vi "tm3samp_06_framerate.vi"() -> ()   [LabVIEW 2023]
panel:
  out "Software FPS":dbl
  out "Camera FPS":dbl
  out "Image":u16[][](graph)
  out "Camera Serial":string
  out "Camera Version":string
  out "Camera Model":string
  out "SMD":dbl
  in  "Scan Mode":dbl min=1.0 max=2.0 step=1.0
  in  "Exposure":dbl min=0.0030207518796992482 max=10.0 step=9.999999747378752e-06
  out "EXP":dbl
  out "SVW":i32
  out "SHW":i32
  out "SVO":i32
  out "SHO":i32
  in  "V Width":i32 min=4 max=2048 step=4
  in  "V Offset":i32 min=0 max=1024 step=4
  in  "H Width":i32 min=4 max=2048 step=4
  in  "H Offset":i32 min=0 max=0 step=4
  in  "Binning":u16(ring) items=["1x1"=1, "2x2"=2, "4x4"=4]
  out "Elapsed Time":u32
  out "Total Frames":i32
  in  "Display":bool=TRUE
  out "error out":errorcluster
  in  "stop":bool
  # "This example displays the frame rate\nof the camera.  Changing the resolution\nof the camera or displaying the images\nwill affect the frame rate."
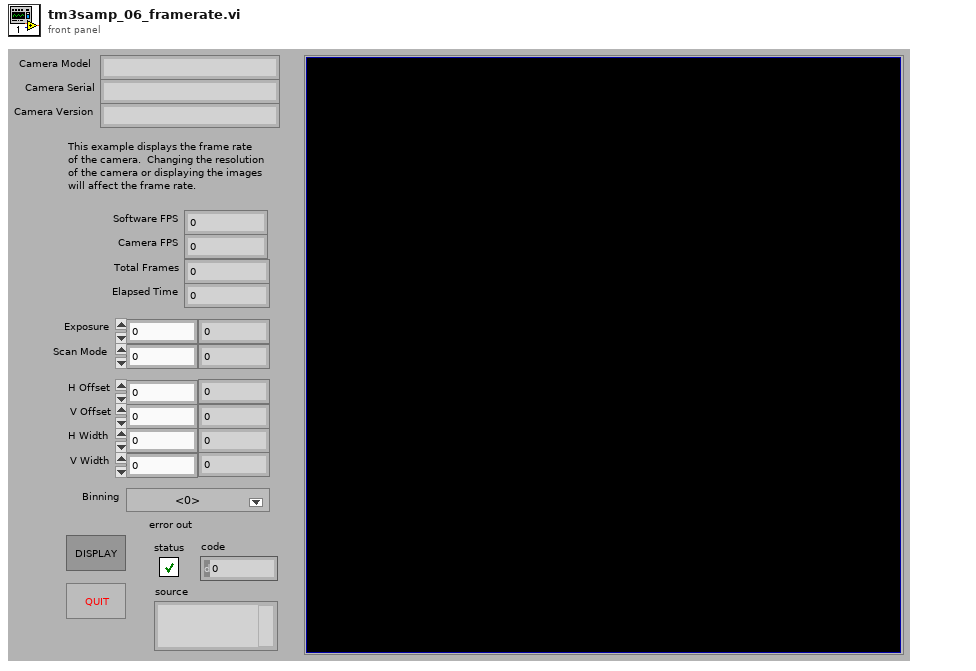
[diagram p1: front panel]
types:
  T1 = cluster{"Model":string, "Camera ID":string, "Firmware":string}
  T2 = cluster{"Value":i32, "Minimum":i32, "Maximum":i32, "Increment":i32}
  T3 = cluster{"height":u32, "width":u32, "datatype":u32}
  T4 = cluster{"H Offset":i32, "V Offset":i32, "H Width":i32, "V Width":i32}
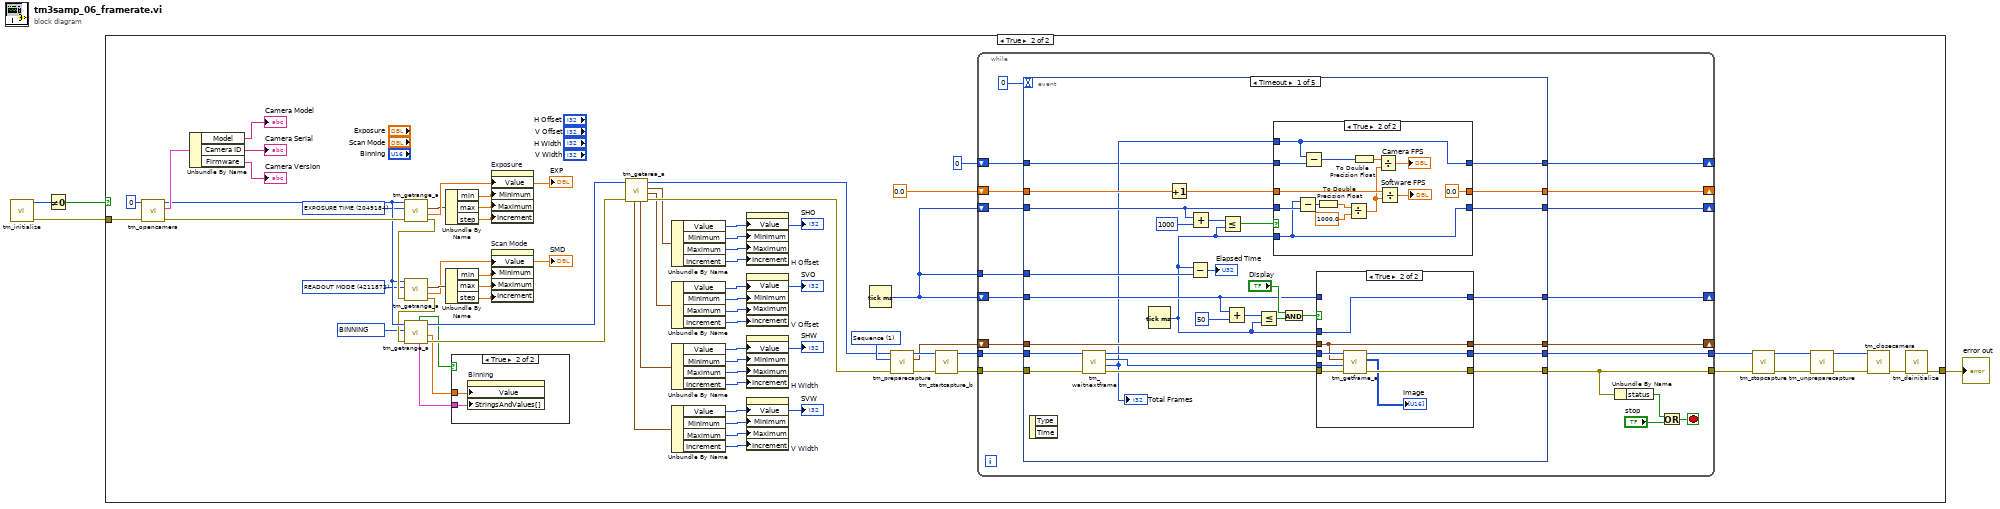
[diagram p0: block diagram]
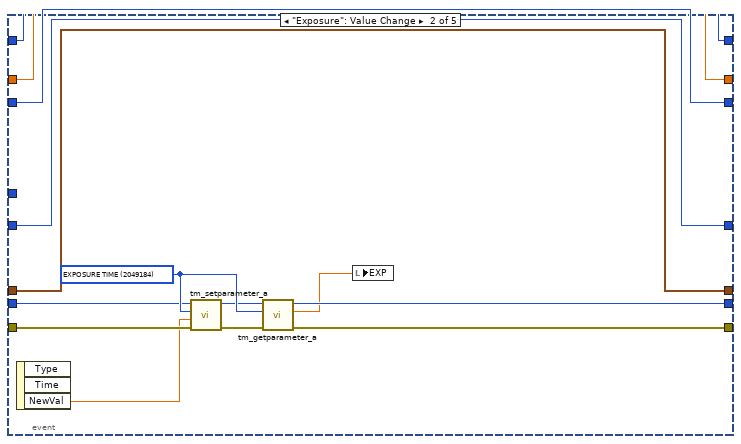
[diagram p6: hidden frame]
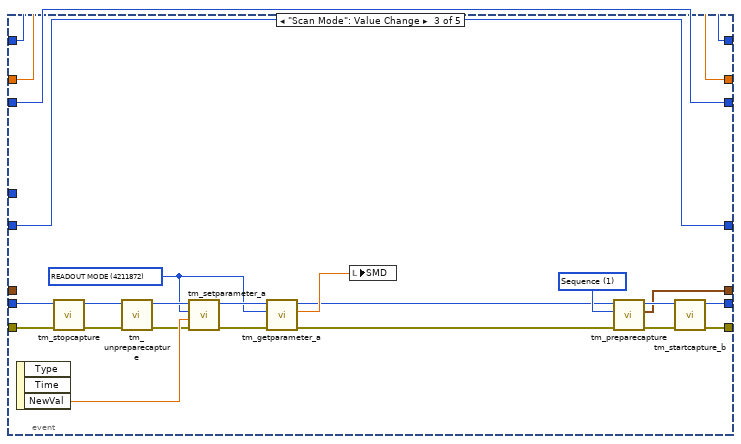
[diagram p7: hidden frame]
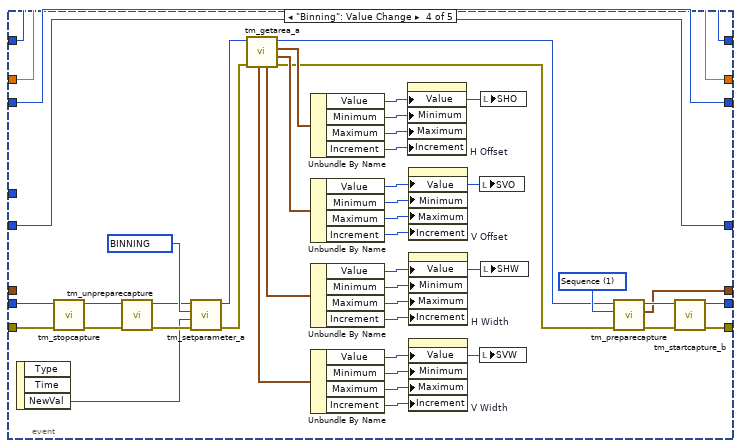
[diagram p8: hidden frame]
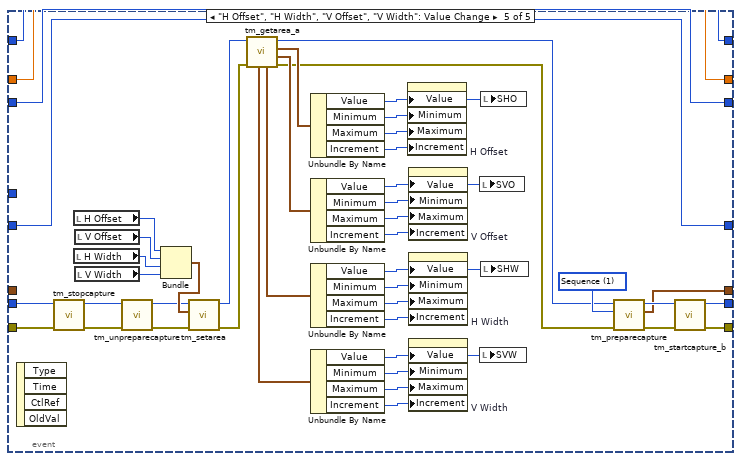
[diagram p9: hidden frame]
diagram:
  n1 = call "tm_initialize.vi"() -> ("error out"=w2:errorcluster, "Number Of Cameras"=w1:u32)  [unwired: 8 in, 2 out]
  n2 = Not Equal To 0?(x=w1) -> (x != 0?=w4:bool)
  n3 = case shown="True" w4 {
    tunnel: [w5 w69] -> w3
    tunnel: w2 -> [w5 w72]
    frame False {
    }
    frame True {
      w6 = u32 2049184 items=["BINNING"=4215968, "BITS PER CHANNEL"=4342976, "ACTIVE VIEW INDEX"=4343136, "CCD MODE"=4212384, "SENSOR MODE"=4212128, "READOUT MODE"=4211872, "EXPOSURE TIME"=2049184, "CONTRAST GAIN"=3163312, "CONTRAST OFFSET"=3163328, "LIGHT MODE"=2114720, "SENSITIVITY"=2114992, "WHITE BALANCE"=3163568, "PHOTON IMAGING MODE"=2115200, "HIGH DYNAMIC RANGE MODE"=3163360, "TRIGGER SOURCE"=1066144, "TRIGGER ACTIVE"=1066160, "TRIGGER MODE"=1066400, "TRIGGER POLARITY"=1066416, "TRIGGER GLOBAL EXPOSURE"=2049680, "FIRST TRIGGER BEHAVIOR"=2049696, "TRIGGER TIMES"=1066448, "OUTPUT TRIGGER POLARITY"=1852592, "OUTPUT TRIGGER DELAY"=1852624, "OUTPUT TRIGGER PERIOD"=1852640, "TEMPERATURE"=2115232, "TEMPERATURE TARGET"=2115264, "SENSOR COOLER FAN"=2115296, "MECHANICAL SHUTTER"=2115488, "BACK FOCUS POSITION"=8422304, "FRAMEBUNDLE MODE"=4346784, "FRAMEBUNDLE NUMBER"=4346800, "LINEBUNDLE HEIGHT"=4212192, "TRIGGER CONNECTOR"=1066432, "IMAGE PIXEL TYPE"=4343296, "OUTPUT TRIGGER KIND"=1852656, "READOUT DIRECTION"=4211904, "CHANNEL SYNC"=1852352] ("Parameter")
      w7 = u32 4211872 items=["BINNING"=4215968, "BITS PER CHANNEL"=4342976, "ACTIVE VIEW INDEX"=4343136, "CCD MODE"=4212384, "SENSOR MODE"=4212128, "READOUT MODE"=4211872, "EXPOSURE TIME"=2049184, "CONTRAST GAIN"=3163312, "CONTRAST OFFSET"=3163328, "LIGHT MODE"=2114720, "SENSITIVITY"=2114992, "WHITE BALANCE"=3163568, "PHOTON IMAGING MODE"=2115200, "HIGH DYNAMIC RANGE MODE"=3163360, "TRIGGER SOURCE"=1066144, "TRIGGER ACTIVE"=1066160, "TRIGGER MODE"=1066400, "TRIGGER POLARITY"=1066416, "TRIGGER GLOBAL EXPOSURE"=2049680, "FIRST TRIGGER BEHAVIOR"=2049696, "TRIGGER TIMES"=1066448, "OUTPUT TRIGGER POLARITY"=1852592, "OUTPUT TRIGGER DELAY"=1852624, "OUTPUT TRIGGER PERIOD"=1852640, "TEMPERATURE"=2115232, "TEMPERATURE TARGET"=2115264, "SENSOR COOLER FAN"=2115296, "MECHANICAL SHUTTER"=2115488, "BACK FOCUS POSITION"=8422304, "FRAMEBUNDLE MODE"=4346784, "FRAMEBUNDLE NUMBER"=4346800, "LINEBUNDLE HEIGHT"=4212192, "TRIGGER CONNECTOR"=1066432, "IMAGE PIXEL TYPE"=4343296, "OUTPUT TRIGGER KIND"=1852656, "READOUT DIRECTION"=4211904, "CHANNEL SYNC"=1852352] ("Parameter")
      w8 = u32 4215968 items=["BINNING"=4215968, "BITS PER CHANNEL"=4342976, "ACTIVE VIEW INDEX"=4343136, "CCD MODE"=4212384, "SENSOR MODE"=4212128, "READOUT MODE"=4211872, "EXPOSURE TIME"=2049184, "CONTRAST GAIN"=3163312, "CONTRAST OFFSET"=3163328, "LIGHT MODE"=2114720, "SENSITIVITY"=2114992, "WHITE BALANCE"=3163568, "PHOTON IMAGING MODE"=2115200, "HIGH DYNAMIC RANGE MODE"=3163360, "TRIGGER SOURCE"=1066144, "TRIGGER ACTIVE"=1066160, "TRIGGER MODE"=1066400, "TRIGGER POLARITY"=1066416, "TRIGGER GLOBAL EXPOSURE"=2049680, "FIRST TRIGGER BEHAVIOR"=2049696, "TRIGGER TIMES"=1066448, "OUTPUT TRIGGER POLARITY"=1852592, "OUTPUT TRIGGER DELAY"=1852624, "OUTPUT TRIGGER PERIOD"=1852640, "TEMPERATURE"=2115232, "TEMPERATURE TARGET"=2115264, "SENSOR COOLER FAN"=2115296, "MECHANICAL SHUTTER"=2115488, "BACK FOCUS POSITION"=8422304, "FRAMEBUNDLE MODE"=4346784, "FRAMEBUNDLE NUMBER"=4346800, "LINEBUNDLE HEIGHT"=4212192, "TRIGGER CONNECTOR"=1066432, "IMAGE PIXEL TYPE"=4343296, "OUTPUT TRIGGER KIND"=1852656, "READOUT DIRECTION"=4211904, "CHANNEL SYNC"=1852352] ("Parameter")
      w67 = 1 items=["Snap", "Sequence"] ("Capture mode")
      n4 = call "tm_opencamera.vi"("error in (no error)"=w72, "Camera Index"=u32 0) -> ("error out"=w21:errorcluster, "Camera Details"=w25:T1, "Handle out"=w15:u32)  [unwired: 7 in]
      n5 = Unbundle By Name(w25) -> ("Model"=→"Camera Model":string, "Camera ID"=→"Camera Serial":string, "Firmware"=→"Camera Version":string)
      n6 = call "tm_getrange_a.vi"("error in (no error)"=w21, "Parameter"=w6, "Handle in"=w15) -> ("error out"=w18:errorcluster, "default"=w20:dbl, "Range"=w19:cluster{"min":dbl, "max":dbl, "step":dbl})  [unwired: 2 in, 4 out]
      "EXP" <- w20
      n7 = call "tm_getrange_a.vi"("error in (no error)"=w18, "Parameter"=w7, "Handle in"=w15) -> ("error out"=w14:errorcluster, "default"=w16:dbl, "Range"=w17:cluster{"min":dbl, "max":dbl, "step":dbl})  [unwired: 2 in, 4 out]
      "SMD" <- w16
      n8 = call "tm_getrange_a.vi"("error in (no error)"=w14, "Parameter"=w8, "Handle in"=w15) -> ("error out"=w13:errorcluster, "default"=w10:dbl, "Handle out"=w12:u32, "Value Names"=w9:cluster{"Name":string, "Value":dbl}[], "Writable"=w11:bool)  [unwired: 2 in, 2 out]
      n9 = Unbundle By Name(w19) -> ("min"=w60:dbl, "max"=w59:dbl, "step"=w58:dbl)
      n10 = Unbundle By Name(w17) -> ("min"=w57:dbl, "max"=w56:dbl, "step"=w55:dbl)
      n11 = case shown="True" w11 {
        tunnel: w9 -> [_ w74]
        tunnel: w10 -> [_ w73]
        frame False {
        }
        frame True {
          n12 = property on="Binning" class="Ring (strict)"("Value"=w73, "StringsAndValues[]"=w74) -> ()  [unwired: 2 in, 2 out]
        }
      }
      n13 = property on="Exposure" class="DigNum (strict)"("Value"=w20, "Minimum"=w60, "Maximum"=w59, "Increment"=w58) -> ()  [unwired: 2 in, 2 out]
      n14 = property on="Scan Mode" class="DigNum (strict)"("Value"=w16, "Minimum"=w57, "Maximum"=w56, "Increment"=w55) -> ()  [unwired: 2 in, 2 out]
      n15 = call "tm_getarea_a.vi"("error in (no error)"=w13, "Handle in"=w12) -> ("error out"=w53:errorcluster, "V Offset"=w52:T2, "H Offset"=w31:T2, "Handle out"=w54:u32, "H Width"=w51:T2, "V Width"=w50:T2)  [unwired: 4 in]
      n16 = Unbundle By Name(w31) -> ("Value"=w30:i32, "Minimum"=w29:i32, "Maximum"=w28:i32, "Increment"=w27:i32)
      "SHO" <- w30
      n17 = Unbundle By Name(w52) -> ("Value"=w40:i32, "Minimum"=w49:i32, "Maximum"=w48:i32, "Increment"=w47:i32)
      "SVO" <- w40
      n18 = Unbundle By Name(w51) -> ("Value"=w39:i32, "Minimum"=w46:i32, "Maximum"=w45:i32, "Increment"=w44:i32)
      "SHW" <- w39
      n19 = Unbundle By Name(w50) -> ("Value"=w38:i32, "Minimum"=w43:i32, "Maximum"=w42:i32, "Increment"=w41:i32)
      "SVW" <- w38
      n20 = property on="H Offset" class="DigNum (strict)"("Value"=w30, "Minimum"=w29, "Maximum"=w28, "Increment"=w27) -> ()  [unwired: 2 in, 2 out]
      n21 = property on="V Offset" class="DigNum (strict)"("Value"=w40, "Minimum"=w49, "Maximum"=w48, "Increment"=w47) -> ()  [unwired: 2 in, 2 out]
      n22 = property on="H Width" class="DigNum (strict)"("Value"=w39, "Minimum"=w46, "Maximum"=w45, "Increment"=w44) -> ()  [unwired: 2 in, 2 out]
      n23 = property on="V Width" class="DigNum (strict)"("Value"=w38, "Minimum"=w43, "Maximum"=w42, "Increment"=w41) -> ()  [unwired: 2 in, 2 out]
      n24 = Tick Count (ms)() -> (millisecond timer value=w61:u32)
      n25 = call "tm_preparecapture.vi"("error in (no error)"=w53, "Capture mode"=w67, "Handle in"=w54) -> ("error out"=w65:errorcluster, "Buffer Info"=w62:T3, "Handle out"=w66:u32)  [unwired: 5 in, 1 out]
      n26 = call "tm_startcapture_b.vi"("error in (no error)"=w65, "Handle in"=w66) -> ("error out"=w64:errorcluster, "Handle out"=w63:u32)  [unwired: 8 in]
      n27 = while {
        tunnel: w64 -> [w82]
        tunnel: [w80] -> w37
        tunnel: [w79] -> w36
        shift-right: [w89] -> _
        shift-left: w61 -> [w87]
        shift-right: [w90] -> _
        shift-left: 0.0 -> [w88]
        shift-right: [w81] -> _
        shift-left: w61 -> [w85]
        tunnel: w63 -> [w83]
        tunnel: w61 -> [w86]
        shift-right: [w78] -> _
        shift-left: w62 -> [w84]
        shift-right: [w75] -> _
        shift-left: 0 -> [w76]
        stop <- w91 stop-if-true
        n28 = event shown="[0] Timeout" {
          selector: _ -> [_ _ _ _ _]
          dyn-events: _ -> [_ _ _ _ _]
          timeout: 0 -> [_ _ _ _ _]
          tunnel: [w98 w164 w187 w223 w268] -> w90
          tunnel: [w97 w165 w188 w224 w269] -> w89
          tunnel: w88 -> [w109 w164 w187 w223 w268]
          tunnel: w87 -> [w100 w165 w188 w224 w269]
          tunnel: w86 -> [w105 _ _ _ _]
          tunnel: w85 -> [w110 w166 w189 w231 w276]
          tunnel: w84 -> [w104 w163 _ _ _]
          tunnel: w83 -> [w112 w158 w184 w200 w238]
          tunnel: w82 -> [w111 w160 w183 w199 w237]
          tunnel: [w108 w166 w189 w231 w276] -> w81
          tunnel: [w107 w155 w178 w226 w271] -> w80
          tunnel: [w106 w153 w179 w227 w272] -> w79
          tunnel: [w103 w163 w177 w225 w270] -> w78
          tunnel: w76 -> [w95 w162 w176 w196 w232]
          tunnel: [w94 w162 w176 w196 w232] -> w75
          event Timeout {
            n29 = event-data() -> ()  [unwired: 1 in, 2 out]
            n30 = call "tm_waitnextframe.vi"("error in (no error)"=w111, "Handle in"=w112) -> ("error out"=w116:errorcluster, "Frame Count"=w96:i32, "Frame Index"=w115:i32, "Handle out"=w117:u32)  [unwired: 6 in]
            "Total Frames" <- w96
            n31 = Tick Count (ms)() -> (millisecond timer value=w102:u32)
            n32 = Increment(x=w109) -> (x+1=w99:dbl)
            n33 = Subtract(x=w102, y=w105) -> (x-y=→"Elapsed Time":u32)
            n34 = Add(x=w100, y=u32 1000) -> (x+y=w123:u32)
            n35 = Less Or Equal?(x=w123, y=w102) -> (x <= y?=w101:bool)
            n36 = Add(x=w110, y=u32 50) -> (x+y=w121:u32)
            n37 = Less Or Equal?(x=w121, y=w102) -> (x <= y?=w119:bool)
            n38 = case shown="True" w101 {
              tunnel: w100 -> [w126 w135]
              tunnel: [w126 w132] -> w97
              tunnel: w99 -> [w125 w138]
              tunnel: w102 -> [_ w132]
              tunnel: [w125 0.0] -> w98
              tunnel: w96 -> [_ w127]
              tunnel: w95 -> [w124 w130]
              tunnel: [w124 w127] -> w94
              frame False {
              }
              frame True {
                n39 = Subtract(x=w132, y=w135) -> (x-y=w134:u32)
                n40 = Subtract(x=w127, y=w130) -> (x-y=w128:i32)
                n41 = To Double Precision Float(number=w134) -> (double precision float=w140:dbl)
                n42 = Divide(x=w140, y=1000.0) -> (x/y=w131:dbl)
                n43 = To Double Precision Float(number=w128) -> (double precision float=w129:dbl)
                n44 = Divide(x=w129, y=w131) -> (x/y=→"Camera FPS":dbl)
                n45 = Divide(x=w138, y=w131) -> (x/y=→"Software FPS":dbl)
              }
            }
            n46 = And(x="Display", y=w119) -> (x .and. y?=w114:bool)
            n47 = case shown="True" w114 {
              tunnel: w110 -> [w144 _]
              tunnel: w102 -> [_ w152]
              tunnel: [w144 w152] -> w108
              tunnel: w117 -> [w143 w151]
              tunnel: w104 -> [w141 w146]
              tunnel: w116 -> [w142 w150]
              tunnel: [w143 w149] -> w107
              tunnel: [w142 w148] -> w106
              tunnel: w115 -> [_ w147]
              tunnel: [w141 w146] -> w103
              frame False {
              }
              frame True {
                n48 = call "tm_getframe_a.vi"("error in (no error)"=w150, "Frame Index"=w147, "Buffer Info"=w146, "Handle in"=w151) -> ("error out"=w148:errorcluster, "Data 16"=→"Image":u16[][], "Handle out"=w149:u32)  [unwired: 3 in, 2 out]
              }
            }
          }
          event "Exposure": Value Change {
            w161 = u32 2049184 items=["SENSOR MODE"=4212128, "CCD MODE"=4212384, "READOUT MODE"=4211872, "ACTIVE VIEW INDEX"=4343136, "BITS PER CHANNEL"=4342976, "IMAGE PIXEL TYPE"=4343296, "BINNING"=4215968, "EXPOSURE TIME"=2049184, "CONTRAST GAIN"=3163312, "CONTRAST OFFSET"=3163328, "LIGHT MODE"=2114720, "SENSITIVITY"=2114992, "PHOTON IMAGING MODE"=2115200, "HIGH DYNAMIC RANGE MODE"=3163360, "WHITE BALANCE"=3163568, "TEMPERATURE"=2115232, "TEMPERATURE TARGET"=2115264, "SENSOR COOLER FAN"=2115296, "LINEBUNDLE HEIGHT"=4212192, "MECHANICAL SHUTTER"=2115488, "BACK FOCUS POSITION"=8422304, "TRIGGER CONNECTOR"=1066432, "TRIGGER SOURCE"=1066144, "OUTPUT TRIGGER SOURCE"=1852576, "TRIGGER GLOBAL EXPOSURE"=2049680, "FIRST TRIGGER BEHAVIOR"=2049696, "CHANNEL SYNC"=1852352, "READOUT DIRECTION"=4211904, "PRE HSYNC COUNT"=1852704] ("Parameter")
            n49 = event-data() -> ("NewVal"=w159:dbl)  [unwired: 1 in, 2 out]
            n50 = call "tm_setparameter_a.vi"("error in (no error)"=w160, "Value in"=w159, "Parameter"=w161, "Handle in"=w158) -> ("error out"=w157:errorcluster, "Handle out"=w156:u32)  [unwired: 6 in]
            n51 = call "tm_getparameter_a.vi"("error in (no error)"=w157, "Parameter"=w161, "Handle in"=w156) -> ("error out"=w153:errorcluster, "Value out"=w154:dbl, "Handle out"=w155:u32)  [unwired: 6 in]
            n52 = local write "EXP"(w154) -> ()
          }
          event "Scan Mode": Value Change {
            w167 = u32 4211872 items=["SENSOR MODE"=4212128, "CCD MODE"=4212384, "READOUT MODE"=4211872, "ACTIVE VIEW INDEX"=4343136, "BITS PER CHANNEL"=4342976, "IMAGE PIXEL TYPE"=4343296, "BINNING"=4215968, "EXPOSURE TIME"=2049184, "CONTRAST GAIN"=3163312, "CONTRAST OFFSET"=3163328, "LIGHT MODE"=2114720, "SENSITIVITY"=2114992, "PHOTON IMAGING MODE"=2115200, "HIGH DYNAMIC RANGE MODE"=3163360, "WHITE BALANCE"=3163568, "TEMPERATURE"=2115232, "TEMPERATURE TARGET"=2115264, "SENSOR COOLER FAN"=2115296, "LINEBUNDLE HEIGHT"=4212192, "MECHANICAL SHUTTER"=2115488, "BACK FOCUS POSITION"=8422304, "TRIGGER CONNECTOR"=1066432, "TRIGGER SOURCE"=1066144, "OUTPUT TRIGGER SOURCE"=1852576, "TRIGGER GLOBAL EXPOSURE"=2049680, "FIRST TRIGGER BEHAVIOR"=2049696, "CHANNEL SYNC"=1852352, "READOUT DIRECTION"=4211904, "PRE HSYNC COUNT"=1852704] ("Parameter")
            w182 = 1 items=["Snap", "Sequence"] ("Capture mode")
            n53 = event-data() -> ("NewVal"=w172:dbl)  [unwired: 1 in, 2 out]
            n54 = call "tm_stopcapture.vi"("error in (no error)"=w183, "Handle in"=w184) -> ("error out"=w185:errorcluster, "Handle out"=w186:u32)  [unwired: 8 in]
            n55 = call "tm_unpreparecapture.vi"("error in (no error)"=w185, "Handle in"=w186) -> ("error out"=w170:errorcluster, "Handle out"=w171:u32)  [unwired: 8 in]
            n56 = call "tm_setparameter_a.vi"("error in (no error)"=w170, "Value in"=w172, "Parameter"=w167, "Handle in"=w171) -> ("error out"=w169:errorcluster, "Handle out"=w168:u32)  [unwired: 6 in]
            n57 = call "tm_getparameter_a.vi"("error in (no error)"=w169, "Parameter"=w167, "Handle in"=w168) -> ("error out"=w175:errorcluster, "Value out"=w174:dbl, "Handle out"=w173:u32)  [unwired: 6 in]
            n58 = local write "SMD"(w174) -> ()
            n59 = call "tm_preparecapture.vi"("error in (no error)"=w175, "Capture mode"=w182, "Handle in"=w173) -> ("error out"=w180:errorcluster, "Buffer Info"=w177:T3, "Handle out"=w181:u32)  [unwired: 5 in, 1 out]
            n60 = call "tm_startcapture_b.vi"("error in (no error)"=w180, "Handle in"=w181) -> ("error out"=w179:errorcluster, "Handle out"=w178:u32)  [unwired: 8 in]
          }
          event "Binning": Value Change {
            w191 = u32 4215968 items=["BINNING"=4215968, "BITS PER CHANNEL"=2, "ACTIVE VIEW INDEX"=3, "CCD MODE"=4, "SENSOR MODE"=5, "READOUT MODE"=6, "EXPOSURE TIME"=7, "CONTRAST GAIN"=8, "CONTRAST OFFSET"=9, "LIGHT MODE"=10, "SENSITIVITY"=11, "WHITE BALANCE"=12, "PHOTON IMAGING MODE"=13, "HIGH DYNAMIC RANGE MODE"=14, "TRIGGER SOURCE"=15, "TRIGGER ACTIVE"=16, "TRIGGER MODE"=17, "TRIGGER POLARITY"=18, "TRIGGER GLOBAL EXPOSURE"=19, "FIRST TRIGGER BEHAVIOR"=20, "TRIGGER TIMES"=21, "OUTPUT TRIGGER POLARITY"=22, "OUTPUT TRIGGER DELAY"=23, "OUTPUT TRIGGER PERIOD"=24, "TEMPERATURE"=25, "TEMPERATURE TARGET"=26, "SENSOR COOLER FAN"=27, "MECHANICAL SHUTTER"=28, "BACK FOCUS POSITION"=29, "FRAMEBUNDLE MODE"=30, "FRAMEBUNDLE NUMBER"=31, "LINEBUNDLE HEIGHT"=32, "TRIGGER CONNECTOR"=33, "IMAGE PIXEL TYPE"=34, "OUTPUT TRIGGER KIND"=35, "READOUT DIRECTION"=36, "CHANNEL SYNC"=37] ("Parameter")
            w230 = 1 items=["Snap", "Sequence"] ("Capture mode")
            n61 = event-data() -> ("NewVal"=w192:u16)  [unwired: 1 in, 2 out]
            n62 = call "tm_stopcapture.vi"("error in (no error)"=w199, "Handle in"=w200) -> ("error out"=w197:errorcluster, "Handle out"=w198:u32)  [unwired: 8 in]
            n63 = call "tm_unpreparecapture.vi"("error in (no error)"=w197, "Handle in"=w198) -> ("error out"=w193:errorcluster, "Handle out"=w190:u32)  [unwired: 8 in]
            n64 = call "tm_setparameter_a.vi"("error in (no error)"=w193, "Value in"=w192, "Parameter"=w191, "Handle in"=w190) -> ("error out"=w194:errorcluster, "Handle out"=w195:u32)  [unwired: 6 in]
            n65 = call "tm_getarea_a.vi"("error in (no error)"=w194, "Handle in"=w195) -> ("error out"=w218:errorcluster, "V Offset"=w220:T2, "H Offset"=w219:T2, "Handle out"=w217:u32, "H Width"=w221:T2, "V Width"=w222:T2)  [unwired: 4 in]
            n66 = Unbundle By Name(w219) -> ("Value"=w213:i32, "Minimum"=w216:i32, "Maximum"=w215:i32, "Increment"=w214:i32)
            n67 = Unbundle By Name(w220) -> ("Value"=w203:i32, "Minimum"=w212:i32, "Maximum"=w211:i32, "Increment"=w210:i32)
            n68 = Unbundle By Name(w221) -> ("Value"=w202:i32, "Minimum"=w209:i32, "Maximum"=w208:i32, "Increment"=w207:i32)
            n69 = Unbundle By Name(w222) -> ("Value"=w201:i32, "Minimum"=w206:i32, "Maximum"=w205:i32, "Increment"=w204:i32)
            n70 = property on="H Offset" class="DigNum (strict)"("Value"=w213, "Minimum"=w216, "Maximum"=w215, "Increment"=w214) -> ()  [unwired: 2 in, 2 out]
            n71 = property on="V Offset" class="DigNum (strict)"("Value"=w203, "Minimum"=w212, "Maximum"=w211, "Increment"=w210) -> ()  [unwired: 2 in, 2 out]
            n72 = property on="H Width" class="DigNum (strict)"("Value"=w202, "Minimum"=w209, "Maximum"=w208, "Increment"=w207) -> ()  [unwired: 2 in, 2 out]
            n73 = property on="V Width" class="DigNum (strict)"("Value"=w201, "Minimum"=w206, "Maximum"=w205, "Increment"=w204) -> ()  [unwired: 2 in, 2 out]
            n74 = local write "SVO"(w203) -> ()
            n75 = local write "SVW"(w201) -> ()
            n76 = local write "SHO"(w213) -> ()
            n77 = local write "SHW"(w202) -> ()
            n78 = call "tm_preparecapture.vi"("error in (no error)"=w218, "Capture mode"=w230, "Handle in"=w217) -> ("error out"=w228:errorcluster, "Buffer Info"=w225:T3, "Handle out"=w229:u32)  [unwired: 5 in, 1 out]
            n79 = call "tm_startcapture_b.vi"("error in (no error)"=w228, "Handle in"=w229) -> ("error out"=w227:errorcluster, "Handle out"=w226:u32)  [unwired: 8 in]
          }
          event "H Offset", "H Width", "V Offset", "V Width": Value Change {
            w275 = 1 items=["Snap", "Sequence"] ("Capture mode")
            n80 = event-data() -> ()  [unwired: 1 in, 4 out]
            n81 = call "tm_stopcapture.vi"("error in (no error)"=w237, "Handle in"=w238) -> ("error out"=w235:errorcluster, "Handle out"=w236:u32)  [unwired: 8 in]
            n82 = local read "H Offset"() -> (w241:i32)
            n83 = local read "H Width"() -> (w242:i32)
            n84 = local read "V Offset"() -> (w243:i32)
            n85 = local read "V Width"() -> (w240:i32)
            n86 = call "tm_unpreparecapture.vi"("error in (no error)"=w235, "Handle in"=w236) -> ("error out"=w233:errorcluster, "Handle out"=w234:u32)  [unwired: 8 in]
            n87 = Bundle("H Offset"=w241, "V Offset"=w243, "H Width"=w242, "V Width"=w240) -> (w239:T4)  [unwired: 1 in]
            n88 = call "tm_setarea.vi"("error in (no error)"=w233, "Sub Region"=w239, "Handle in"=w234) -> ("error out"=w244:errorcluster, "Handle out"=w245:u32)  [unwired: 7 in]
            n89 = call "tm_getarea_a.vi"("error in (no error)"=w244, "Handle in"=w245) -> ("error out"=w263:errorcluster, "V Offset"=w265:T2, "H Offset"=w264:T2, "Handle out"=w262:u32, "H Width"=w266:T2, "V Width"=w267:T2)  [unwired: 4 in]
            n90 = Unbundle By Name(w264) -> ("Value"=w258:i32, "Minimum"=w261:i32, "Maximum"=w260:i32, "Increment"=w259:i32)
            n91 = Unbundle By Name(w265) -> ("Value"=w248:i32, "Minimum"=w257:i32, "Maximum"=w256:i32, "Increment"=w255:i32)
            n92 = Unbundle By Name(w266) -> ("Value"=w247:i32, "Minimum"=w254:i32, "Maximum"=w253:i32, "Increment"=w252:i32)
            n93 = Unbundle By Name(w267) -> ("Value"=w246:i32, "Minimum"=w251:i32, "Maximum"=w250:i32, "Increment"=w249:i32)
            n94 = property on="H Offset" class="DigNum (strict)"("Value"=w258, "Minimum"=w261, "Maximum"=w260, "Increment"=w259) -> ()  [unwired: 2 in, 2 out]
            n95 = property on="V Offset" class="DigNum (strict)"("Value"=w248, "Minimum"=w257, "Maximum"=w256, "Increment"=w255) -> ()  [unwired: 2 in, 2 out]
            n96 = property on="H Width" class="DigNum (strict)"("Value"=w247, "Minimum"=w254, "Maximum"=w253, "Increment"=w252) -> ()  [unwired: 2 in, 2 out]
            n97 = property on="V Width" class="DigNum (strict)"("Value"=w246, "Minimum"=w251, "Maximum"=w250, "Increment"=w249) -> ()  [unwired: 2 in, 2 out]
            n98 = local write "SVO"(w248) -> ()
            n99 = local write "SVW"(w246) -> ()
            n100 = local write "SHO"(w258) -> ()
            n101 = local write "SHW"(w247) -> ()
            n102 = call "tm_preparecapture.vi"("error in (no error)"=w263, "Capture mode"=w275, "Handle in"=w262) -> ("error out"=w273:errorcluster, "Buffer Info"=w270:T3, "Handle out"=w274:u32)  [unwired: 5 in, 1 out]
            n103 = call "tm_startcapture_b.vi"("error in (no error)"=w273, "Handle in"=w274) -> ("error out"=w272:errorcluster, "Handle out"=w271:u32)  [unwired: 8 in]
          }
        }
        n104 = Unbundle By Name(w79) -> ("status"=w92:bool)
        n105 = Or(x=w92, y="stop") -> (x .or. y?=w91:bool)
      }
      n106 = call "tm_stopcapture.vi"("error in (no error)"=w36, "Handle in"=w37) -> ("error out"=w33:errorcluster, "Handle out"=w34:u32)  [unwired: 8 in]
      n107 = call "tm_unpreparecapture.vi"("error in (no error)"=w33, "Handle in"=w34) -> ("error out"=w32:errorcluster, "Handle out"=w35:u32)  [unwired: 8 in]
      n108 = call "tm_closecamera.vi"("error in (no error)"=w32, "Handle in"=w35) -> ("error out"=w70:errorcluster)  [unwired: 9 in]
      n109 = call "tm_deinitialize.vi"("error in (no error)"=w70) -> ("error out"=w69:errorcluster)  [unwired: 10 in]
    }
  }
  "error out" <- w3
